vi "Get Buffer Size.vi"(8 "error in (no error)":errorcluster, 11 "Logger in.lvclass":refnum<class "Logger.lvclass">) -> (0 "error out":errorcluster, 2 "Buffer Size":i32, 3 "Logger out.lvclass":refnum<class "Logger.lvclass">)   [LabVIEW 2017, in "Logger.lvclass"]
uses:
  Logger.lvclass
  Logger.lvclass/Logger.ctl
  <vilib>/Waveform/WDTOps.llb/WDT Number of Waveform Samples DBL.vi
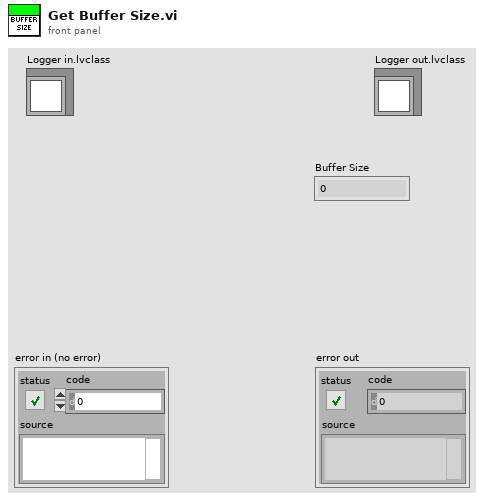
[diagram p1: front panel]
types:
  T1 = cluster{"Tag Units":string, "Tag Path":string, "Waveform":waveform(dbl), "Log":bool, "Tag Reference":refnum<class "NI Skyline Tag.lvclass">}[]
  T2 = cluster{"Tag Units":string, "Tag Path":string, "Waveform":waveform(dbl), "Log":bool, "Tag Reference":refnum<class "NI Skyline Tag.lvclass">}
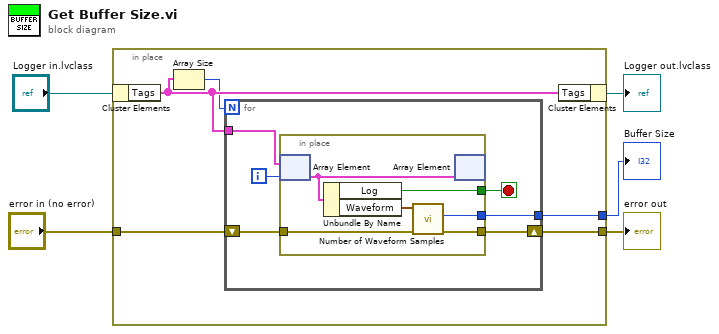
[diagram p0: block diagram]
diagram:
  n1 = in-place {
    in-place-border: "error in (no error)" -> [w10]
    in-place-border: [w9] -> w4
    in-place-border: [w8] -> w3
    n2 = in-place-cluster #1("Logger in.lvclass") -> ("Tags"=w7:T1)
    n3 = Array Size(array=w7) -> (size(s)=w6:i32)
    n4 = for {
      N: w6 -> [_]
      tunnel: w7 -> [w11]
      shift-right: [w15] -> w9
      shift-left: w10 -> [w16]
      tunnel: [w13] -> w8
      i -> [w12]
      stop <- w14 stop-if-true
      n5 = in-place {
        in-place-border: w16 -> [w22]
        in-place-border: [w21] -> w15
        in-place-border: [w19] -> w14
        in-place-border: [w18] -> w13
        n6 = in-place-array #2(w11, w12) -> (w17:T2)
        n7 = Unbundle By Name(w17) -> ("Log"=w19:bool, "Waveform"=w20:waveform(dbl))
        n8 = call-poly <vilib>:"Number of Waveform Samples.vi"("error in (no error)"=w22, "waveform in"=w20) -> ("error out"=w21:errorcluster, "number of samples"=w18:i32)  [unwired: 7 in, 1 out]
        n9 = in-place-array #2(w17) -> ()  [unwired: 2 out]
      }
    }
    n10 = in-place-cluster #1("Tags"=w7) -> (→"Logger out.lvclass":refnum<class "Logger.lvclass">)
  }
  "error out" <- w4
  "Buffer Size" <- w3
